vi "CalculateWallPose.vi"(8 "Lidar Angles":dbl[](array[numeric])=[-99.9609375, -99.609375, -99.2578125, -98.90625, -98.5546875, -98.203125, -97.8515625, -97.5, -97.1484375, -96.796875, -96.4453125, -96.09375, -95.7421875, -95.390625, -95.0390625, -94.6875, -94.3359375, -93.984375, -93.6328125, -93.28125, -92.9296875, -92.578125, -92.2265625, -91.875, -91.5234375, -91.171875, -90.8203125, -90.46875, -90.1171875, -89.765625, -89.4140625, -89.0625, -88.7109375, -88.359375, -88.0078125, -87.65625, -87.3046875, -86.953125, -86.6015625, -86.25, -85.8984375, -85.546875, -85.1953125, -84.84375, -84.4921875, -84.140625, -83.7890625, -83.4375, -83.0859375, -82.734375, -82.3828125, -82.03125, -81.6796875, -81.328125, -80.9765625, -80.625, -80.2734375, -79.921875, -79.5703125, -79.21875, -78.8671875, -78.515625, -78.1640625, -77.8125, -77.4609375, -77.109375, -76.7578125, -76.40625, -76.0546875, -75.703125, -75.3515625, -75.0, -74.6484375, -74.296875, -73.9453125, -73.59375, -73.2421875, -72.890625, -72.5390625, -72.1875, -71.8359375, -71.484375, -71.1328125, -70.78125, -70.4296875, -70.078125, -69.7265625, -69.375, -69.0234375, -68.671875, -68.3203125, -67.96875, -67.6171875, -67.265625, -66.9140625, -66.5625, -66.2109375, -65.859375, -65.5078125, -65.15625, -64.8046875, -64.453125, -64.1015625, -63.75, -63.3984375, -63.046875, -62.6953125, -62.34375, -61.9921875, -61.640625, -61.2890625, -60.9375, -60.5859375, -60.234375, -59.8828125, -59.53125, -59.1796875, -58.828125, -58.4765625, -58.125, -57.7734375, -57.421875, -57.0703125, -56.71875, -56.3671875, -56.015625, -55.6640625, -55.3125, -54.9609375, -54.609375, -54.2578125, -53.90625, -53.5546875, -53.203125, -52.8515625, -52.5, -52.1484375, -51.796875, -51.4453125, -51.09375, -50.7421875, -50.390625, -50.0390625, -49.6875, -49.3359375, -48.984375, -48.6328125, -48.28125, -47.9296875, -47.578125, -47.2265625, -46.875, -46.5234375, -46.171875, -45.8203125, -45.46875, -45.1171875], 9 "Lidar Magnitude":dbl[](array[numeric])=[372.0, 372.0, 372.0, 372.0, 372.0, 373.0, 372.0, 371.0, 373.0, 371.0, 371.0, 371.0, 378.0, 375.0, 377.0, 380.0, 380.0, 377.0, 378.0, 378.0, 376.0, 370.0, 373.0, 372.0, 369.0, 369.0, 371.0, 371.0, 371.0, 372.0, 372.0, 378.0, 372.0, 371.0, 371.0, 370.0, 370.0, 370.0, 369.0, 369.0, 369.0, 369.0, 369.0, 369.0, 376.0, 376.0, 376.0, 366.0, 375.0, 366.0, 371.0, 371.0, 375.0, 372.0, 375.0, 378.0, 378.0, 378.0, 378.0, 378.0, 376.0, 375.0, 375.0, 375.0, 378.0, 378.0, 378.0, 378.0, 378.0, 380.0, 380.0, 378.0, 377.0, 377.0, 377.0, 377.0, 377.0, 378.0, 382.0, 382.0, 383.0, 383.0, 383.0, 383.0, 387.0, 387.0, 387.0, 387.0, 387.0, 388.0, 389.0, 391.0, 393.0, 393.0, 393.0, 396.0, 398.0, 398.0, 399.0, 399.0, 399.0, 399.0, 400.0, 399.0, 400.0, 401.0, 401.0, 403.0, 405.0, 405.0, 406.0, 406.0, 412.0, 411.0, 412.0, 413.0, 421.0, 414.0, 419.0, 419.0, 419.0, 419.0, 424.0, 424.0, 426.0, 433.0, 429.0, 429.0, 433.0, 429.0, 429.0, 436.0, 437.0, 442.0, 443.0, 443.0, 449.0, 451.0, 451.0, 451.0, 457.0, 459.0, 457.0, 459.0, 460.0, 465.0, 467.0, 472.0, 472.0, 478.0, 478.0, 478.0, 479.0, 485.0, 485.0, 485.0, 496.0]) -> (0 "Angle to Wall":dbl, 1 "Distance to Wall":dbl=368.4, 2 "Can't see wall":bool, 3 "OH SHIT NO LIDAR DATA!!!":bool)   [LabVIEW 2017]
uses:
  <vilib>/Analysis/NI_AALPro.lvlib
panel:
  out "regression error":dbl
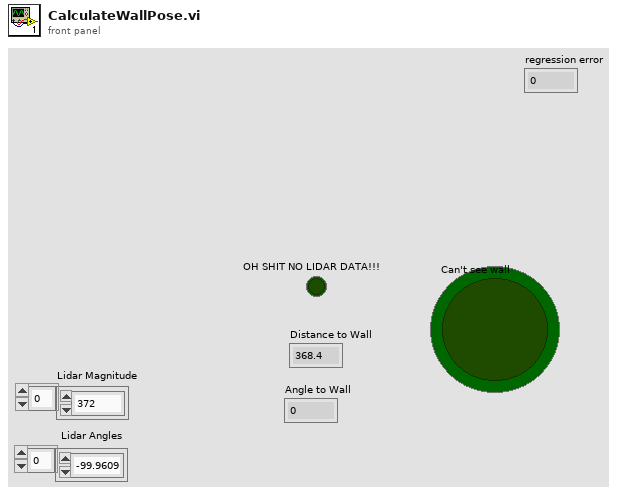
[diagram p1: front panel]
types:
  T1 = cluster{"slope min":dbl, "slope max":dbl, "intercept min":dbl, "intercept max":dbl}
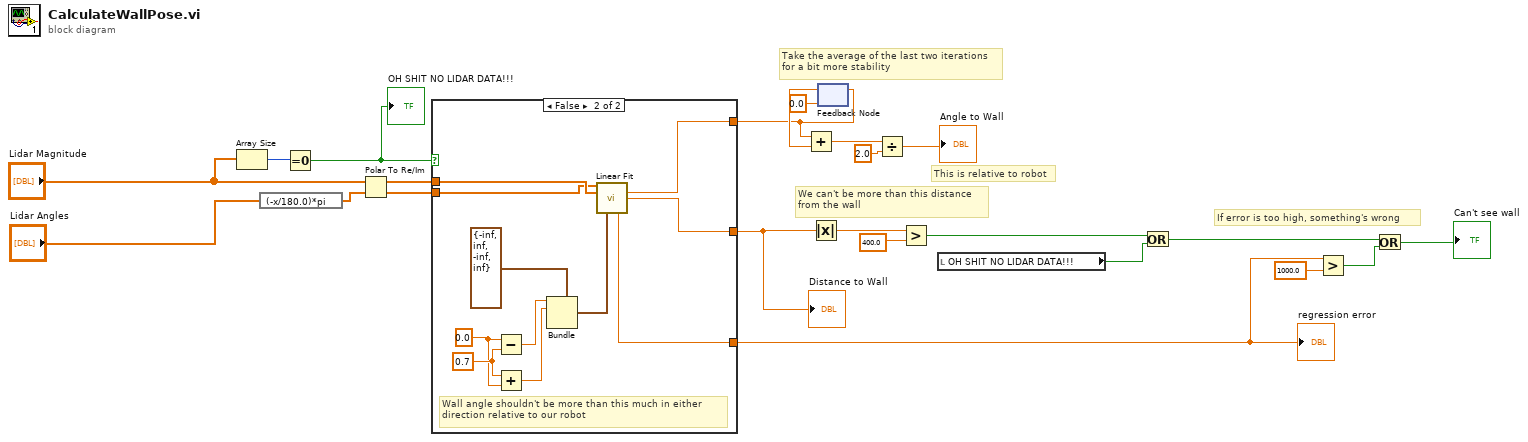
[diagram p0: block diagram]
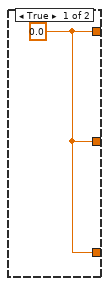
[diagram p2: hidden frame]
diagram:
  # "If error is too high, something's wrong"
  # "We can't be more than this distance\nfrom the wall"
  # "Take the average of the last two iterations\nfor a bit more stability"
  # "This is relative to robot"
  n1 = Array Size(array="Lidar Magnitude") -> (size(s)=w19:i32)
  n2 = expression code="(-x/180.0)*pi" ("degrees to radians")("Lidar Angles") -> (w23:dbl[])
  n3 = Equal To 0?(x=w19) -> (x = 0?=w6:bool)
  "OH SHIT NO LIDAR DATA!!!" <- w6
  n4 = Polar To Re/Im(2:w23, 3:"Lidar Magnitude") -> (0:w20:dbl[], 1:w21:dbl[])
  n5 = case shown="False" w6 {
    tunnel: w21 -> [_ w35]
    tunnel: w20 -> [_ w34]
    tunnel: [w24 w33] -> w13
    tunnel: [w24 w32] -> w8
    tunnel: [w24 w25] -> w11
    frame True {
      w24 = 0.0 ("slope")
    }
    frame False {
      w26 = 0.0 ("y")
      w30 = 0.7 ("y")
      # "Wall angle shouldn't be more than this much in either\ndirection relative to our robot"
      n6 = Subtract(x=w26, y=w30) -> (x-y=w29:dbl)
      n7 = Add(x=w30, y=w26) -> (x+y=w28:dbl)
      n8 = Bundle(cluster=T1 {"slope min"=-inf, "slope max"=inf, "intercept min"=-inf, "intercept max"=inf} ("parameter bounds"), "slope min"=w29, "slope max"=w28) -> (w27:T1)  [unwired: 2 in]
      n9 = call <vilib>:"Linear Fit.vi"("Y"=w34, "X"=w35, "parameter bounds"=w27) -> ("slope"=w33:dbl, "intercept"=w32:dbl, "residue"=w25:dbl)  [unwired: 8 in, 2 out]
    }
  }
  "Distance to Wall" <- w8
  "regression error" <- w11
  n10 = Absolute Value(x=w8) -> (abs(x)=w7:dbl)
  n11 = feedback-in #1(w13) -> ()
  n12 = feedback #1(0.0 ("slope")) -> (w14:dbl)
  n13 = Add(x=w13, y=w14) -> (x+y=w16:dbl)
  n14 = Divide(x=w16, y=2.0) -> (x/y=→"Angle to Wall":dbl)
  n15 = Greater?(x=w7, y=400.0) -> (0:w5:bool)
  n16 = local read "OH SHIT NO LIDAR DATA!!!"() -> (w4:bool)
  n17 = Or(x=w5, y=w4) -> (x .or. y?=w3:bool)
  n18 = Greater?(x=w11, y=1000.0) -> (0:w2:bool)
  n19 = Or(x=w3, y=w2) -> (x .or. y?=→"Can't see wall":bool)
